vi "Configure High Amplitude.vi"(6 "channel":i32=1 min=1 max=4, 8 "error in (no error)":errorcluster, 10 "amplitude (V)":dbl=0.005 min=0.005 max=5.0, 11 "VISA resource name":refnum<visa-resource-name>) -> (0 "error out":errorcluster, 3 "VISA resource name out":refnum<visa-resource-name>)   [LabVIEW 2019, in "Pulse Rider PG-1000.lvlib"]
doc: "This command sets the high level of the output amplitude for the specified channel\n\namplitude: the amplitude in V\nchannel: the output channel int from 1 to 4"
uses:
  <instrlib>/LV_PulseRiderPG1000/Pulse Rider PG-1000.lvlib
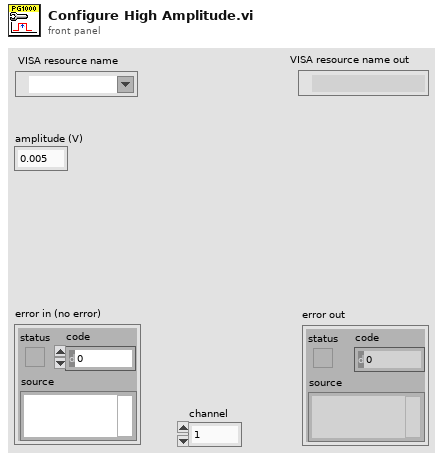
[diagram p1: front panel]
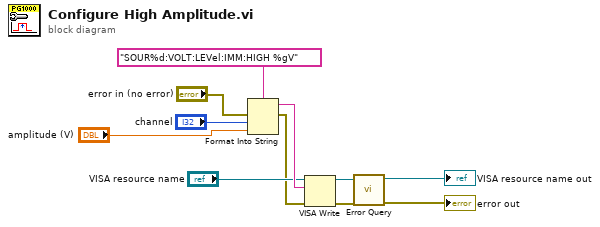
[diagram p0: block diagram]
diagram:
  n1 = Format Into String(format string="SOUR%d:VOLT:LEVel:IMM:HIGH %gV", error in="error in (no error)", "channel", "amplitude (V)") -> (resulting string=w8:string, error out=w2:errorcluster)  [unwired: 1 in]
  n2 = VISA Write(VISA resource name="VISA resource name", write buffer=w8, error in (no error)=w2) -> (VISA resource name out=w11:refnum<visa-resource-name>, error out=w10:errorcluster)  [unwired: 1 out]
  n3 = call <instrlib>:"Error Query.vi"("error in (no error)"=w10, "VISA resource name"=w11) -> ("error out"=→"error out":errorcluster, "VISA resource name out"=→"VISA resource name out":refnum<visa-resource-name>)  [unwired: 6 in, 2 out]
